vi "Read Public Thread Error.vi"(8 "error in (no error)":errorcluster, 10 "public thread index":i32, 11 "Thread Manager in":refnum<class "Thread Manager.lvclass">) -> (0 "error out":errorcluster, 2 "thread error":errorcluster, 3 "Thread Manager out":refnum<class "Thread Manager.lvclass">)   [LabVIEW 2021, in "DSF Core.lvlib" / "Thread Manager.lvclass"]
uses:
  Thread Manager.lvclass
  Thread Manager.lvclass/Thread Manager.ctl
  Thread/Thread.lvclass/Thread.ctl
  Pointers/Error/Error Pointer.lvclass/Error Pointer.ctl
  <vilib>/NI/Memory Manager/Classes/Pointer/Pointer.lvclass/Pointer.ctl
  Pointers/Error/Read Error Pointer.vi
  <vilib>/Utility/error.llb/Clear Errors.vi
  <vilib>/NI/Memory Manager/Classes/Pointer/Read.vi
  <vilib>/NI/Memory Manager/Classes/Pointer/Read 1D U8.vi
  Thread/Logging/Trim Error Whitespace.vi
  Pointers/Error/Get Power Of 2.vi
  <vilib>/NI/Memory Manager/Classes/Pointer/Read (No Check).vi
  <vilib>/NI/Memory Manager/Classes/Pointer/Read (No Check) 1D U8.vi
  <vilib>/NI/Memory Manager/Classes/Pointer/Check Move.vi
  <vilib>/NI/Memory Manager/Classes/Pointer/Get Address.vi
  <vilib>/NI/Memory Manager/Classes/Pointer/Check Null Pointer.vi
  <vilib>/NI/Memory Manager/Classes/Pointer/Check Count.vi
  <vilib>/NI/Memory Manager/Classes/Pointer/Check Bounds (Power of 2).vi
  <vilib>/NI/Memory Manager/Classes/Pointer/Errors.vi
  <vilib>/NI/Memory Manager/Classes/Pointer/Null Pointer.vi
  <vilib>/NI/Memory Manager/Classes/Pointer/Is Null.vi
  <vilib>/NI/Memory Manager/Classes/Pointer/Get Size.vi
  <vilib>/NI/Memory Manager/Classes/Pointer/Out of Bounds.vi
  <vilib>/NI/Memory Manager/Classes/Pointer/Check Bounds.vi
  <vilib>/NI/Memory Manager/Classes/Pointer/Create Error.vi
  <vilib>/NI/Memory Manager/VIs/Write String to Source.vi
  <vilib>/NI/Memory Manager/Classes/Pointer/Write Pointer Size to Error.vi
  <vilib>/NI/Memory Manager/VIs/Write Numeric to Source.vi
  <vilib>/NI/Memory Manager/VIs/Write Numeric Scalar to Source (Base10 U64).vi
  <vilib>/NI/Memory Manager/Classes/Pointer/Check Bounds (Pointer).vi
  <vilib>/NI/Memory Manager/Classes/Pointer/Check Bounds (Buffer).vi
  <vilib>/NI/Memory Manager/VIs/New Error Cluster.vi
  <vilib>/NI/Memory Manager/VIs/New Error Cluster (512B).vi
  <vilib>/NI/Memory Manager/VIs/Set Error Status.vi
  <vilib>/NI/Memory Manager/VIs/Set Error Code.vi
  <vilib>/NI/Memory Manager/VIs/Set Error Source.vi
  <vilib>/NI/Memory Manager/Constants/Constants.vi
  <vilib>/NI/Memory Manager/Constants/Library Name.vi
  <vilib>/NI/Memory Manager/Classes/Pointer/Pointer Error Info.vi
  <vilib>/NI/Memory Manager/Constants/Pointer Class Name.vi
  <vilib>/NI/Memory Manager/Classes/Pointer/Buffer Underflow.vi
  Pointers/Error/Error Pointer.lvclass
  C:/Program Files/National Instruments/LabVIEW 2021/vi.lib/NI/Memory Manager/Classes/Pointer/Pointer.lvclass
  Thread/Thread.lvclass
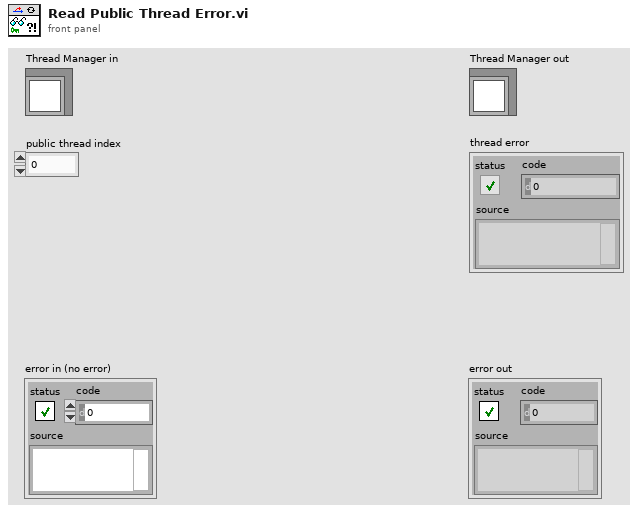
[diagram p1: front panel]
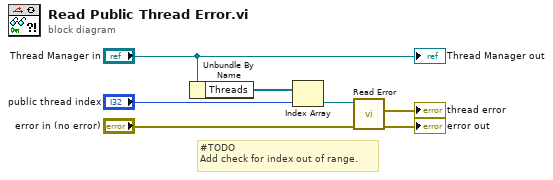
[diagram p0: block diagram]
diagram:
  # "#TODO\nAdd check for index out of range."
  n1 = Unbundle By Name("Thread Manager in") -> ("Threads"=w6:refnum<class "Thread.lvclass">[])
  n2 = Index Array(array=w6, index="public thread index") -> (element=w4:refnum<class "Thread.lvclass">)
  n3 = call "Read Error.vi"("error in (no error)"="error in (no error)", "Thread in"=w4) -> ("error out"=→"error out":errorcluster, "error"=→"thread error":errorcluster)  [unwired: 7 in, 1 out]
  "Thread Manager out" <- "Thread Manager in"
